vi "ROI and SWC editing tool.vi"() -> ()   [LabVIEW 2017]
panel:
  in  "Stop Button":bool
  in  "Open ROI data file":bool
  in  "Tab Control":T1(tab)
  in  "ROI":i32(listbox)
  in  "SWC":i32(listbox)
  out "ROI.dat file":path
  out "SWC File":path
  out "ROI":string[][](array[string])
  out "error out":errorcluster
  in  "error in":errorcluster
  in  "file path (use dialog)":path
  in  "Top rows to delete":i32=5
  out "number":dbl[][](array[numeric])
  out "x-y":dbl[](array[numeric])
  out "dmotorZ":dbl[](array[numeric])
  out "daolZ":dbl[](array[numeric])
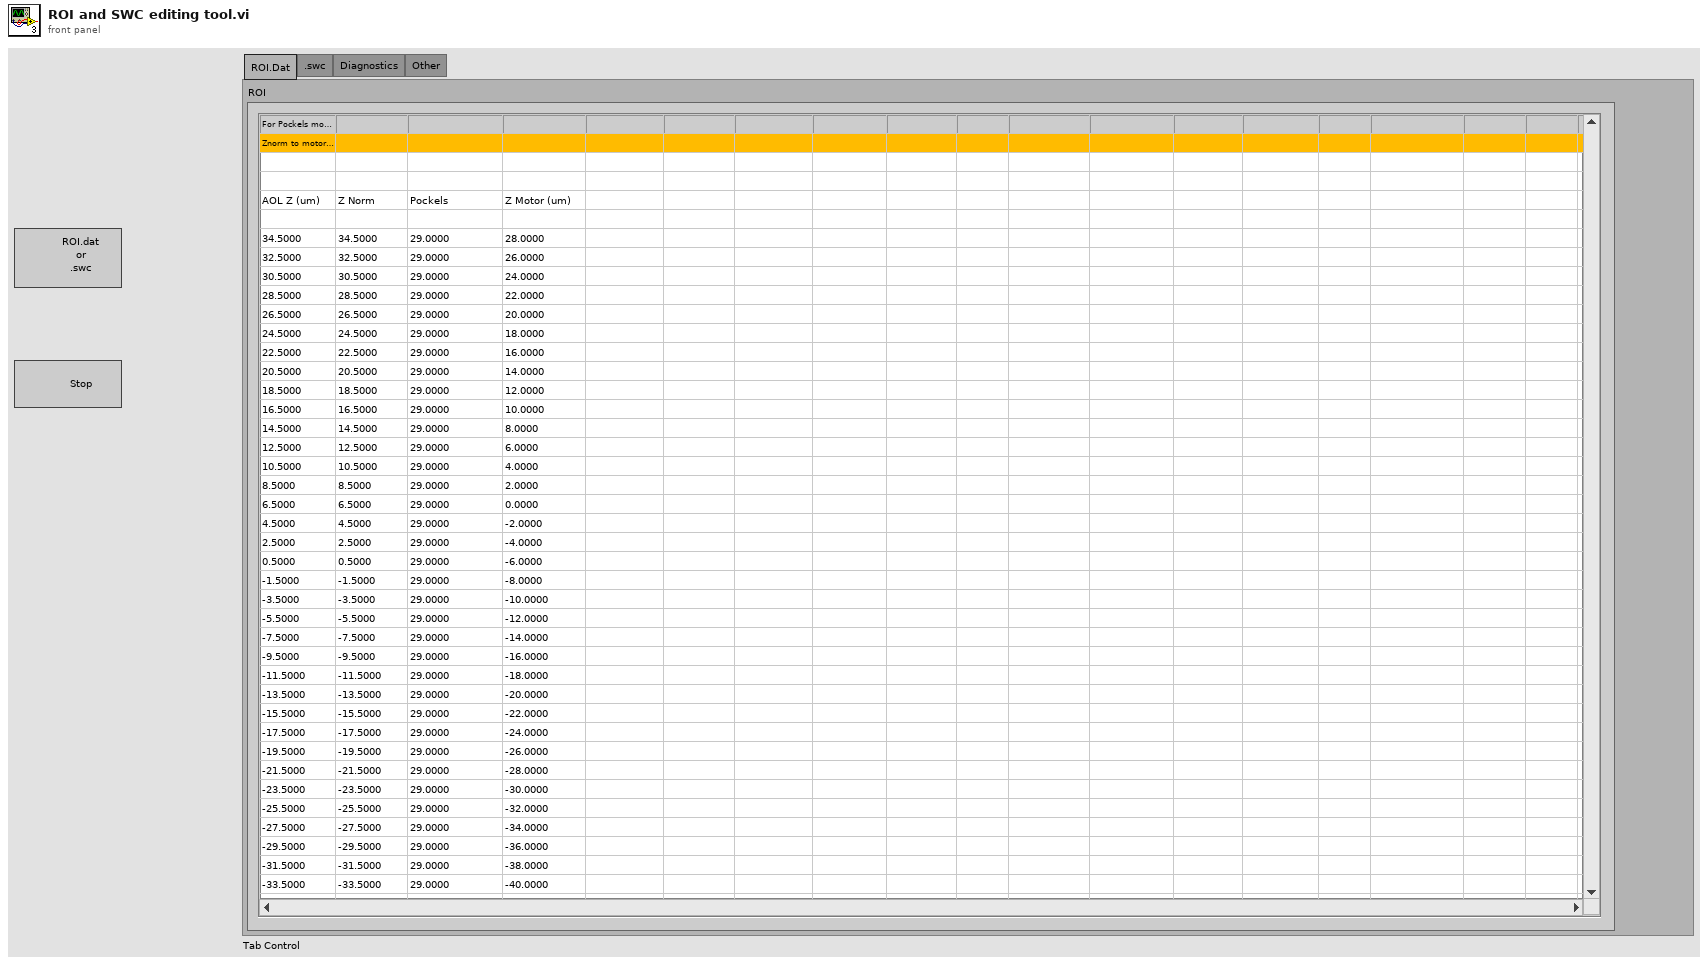
[diagram p1: front panel]
types:
  T1 = enum32{"ROI.Dat", ".swc", "Diagnostics", "Other"}
  T2 = enum16{"open", "replace", "create", "open or create", "replace or create", "replace or create with confirmation"}
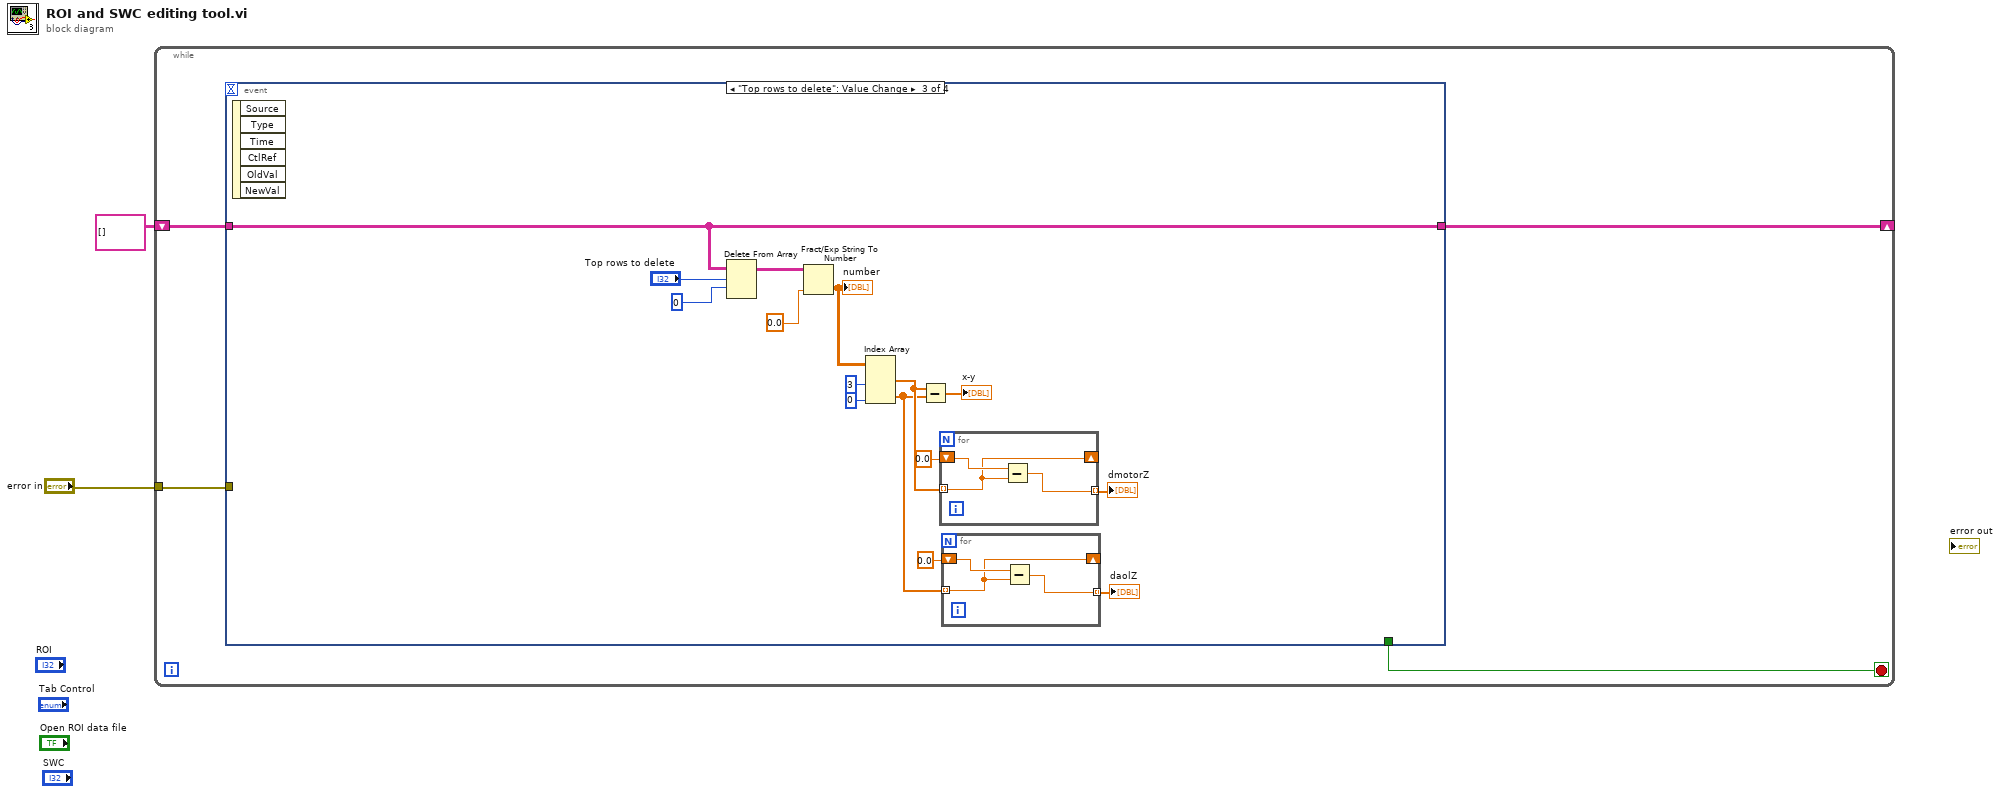
[diagram p0: block diagram]
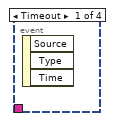
[diagram p2: hidden frame]
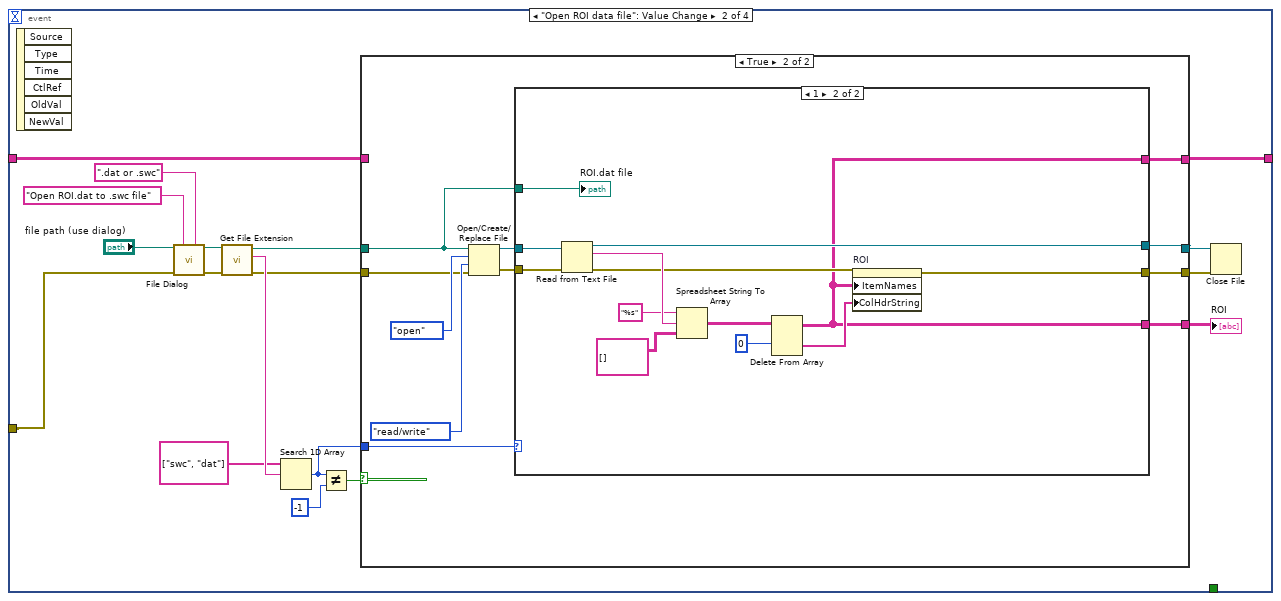
[diagram p3: hidden frame]
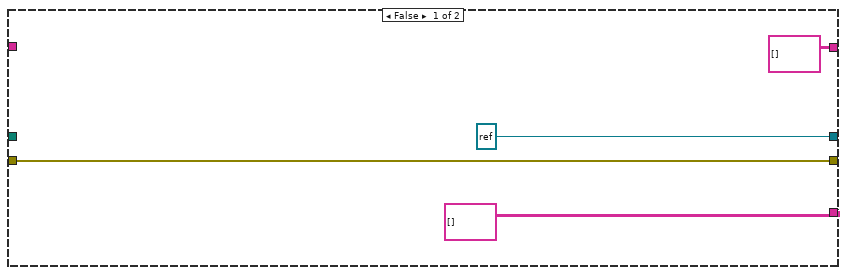
[diagram p4: hidden frame]
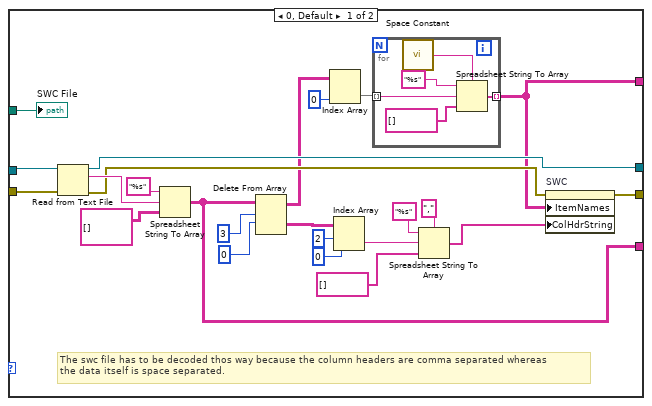
[diagram p5: hidden frame]
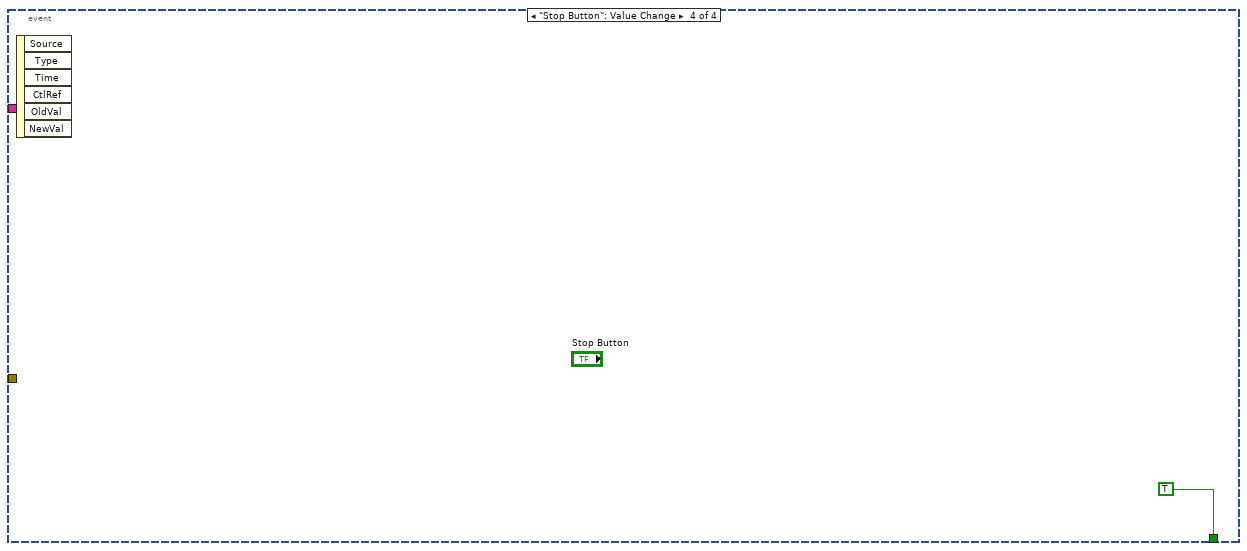
[diagram p6: hidden frame]
diagram:
  n1 = while {
    tunnel: "error in" -> [w6]
    shift-right: [w4] -> _
    shift-left: string[][] [] -> [w3]
    stop <- w5 stop-if-true
    n2 = event shown="[2] \"Top rows to delete\": Value Change" {
      selector: _ -> [_ _ _ _]
      dyn-events: _ -> [_ _ _ _]
      timeout: _ -> [_ _ _ _]
      tunnel: w6 -> [_ w9 _ _]
      tunnel: [_ _ _ TRUE] -> w5
      tunnel: [_ w8 w93 _] -> w4
      tunnel: w3 -> [_ w7 w93 _]
      event Timeout {
        n3 = event-data() -> ()  [unwired: 1 in, 3 out]
      }
      event "Open ROI data file": Value Change {
        n4 = event-data() -> ()  [unwired: 1 in, 6 out]
        n5 = call "File Dialog"("start path"="file path (use dialog)", "prompt"="Open ROI.dat to .swc file", "button label"=".dat or .swc" ("prompt"), "error in"=w9) -> ("selected path"=w16:path, "error out"=w15:errorcluster)  [unwired: 8 in, 2 out]
        n6 = call <vilib>:"Get File Extension.vi"("error in (no error)"=w15, "file"=w16) -> ("error out"=w17:errorcluster, "lowercase file extension"=w22:string, "dup file"=w18:path)  [unwired: 5 in, 2 out]
        n7 = Search 1D Array(1D array=string[] ["swc", "dat"], element=w22) -> (index of element=w24:i32)  [unwired: 1 in]
        n8 = Not Equal?(x=w24, y=-1) -> (x != y?=w23:bool)
        n9 = case shown="True" w23 {
          tunnel: w17 -> [w27 w37]
          tunnel: w18 -> [_ w30]
          tunnel: [string[][] [] w36] -> w19
          tunnel: [w27 w35] -> w20
          tunnel: [refnum<file> refnum ("refnum out") w31] -> w21
          tunnel: w24 -> [_ w34]
          tunnel: [string[][] [] w29] -> w8
          tunnel: w7 -> [_ _]
          frame False {
          }
          frame True {
            n10 = Open/Create/Replace File(file path (use dialog)=w30, error in=w37, operation (0:open)=T2."open", access (0:read/write)=enum16{"read/write", "read-only", "write-only"}."read/write") -> (refnum out=w32:refnum<file>, error out=w33:errorcluster)  [unwired: 2 in, 1 out]
            n11 = case shown="1" w34 {
              tunnel: [w48 w69] -> w36
              tunnel: [w63 w79] -> w35
              tunnel: w33 -> [w62 w75]
              tunnel: w32 -> [w61 w74]
              tunnel: [w49 w71] -> w31
              tunnel: w30 -> [w41 w70]
              tunnel: [w40 w69] -> w29
              frame 0, Default {
                # "The swc file has to be decoded thos way because the column headers are comma separated whereas\nthe data itself is space separated."
                n12 = Read from Text File(file (use dialog)=w61, error in=w62) -> (refnum out=w49:refnum<file>, text=w59:string, error out=w50:errorcluster)  [unwired: 2 in, 1 out]
                n13 = Spreadsheet String To Array(format string="%s", spreadsheet string=w59, array type (2D Dbl)=string[][] []) -> (array=w48:string[][])  [unwired: 1 in]
                n14 = Delete From Array(array=w48, length=3, index (row)=0 ("index")) -> (deleted portion=w55:string[][], array with subset deleted=w44:string[][])  [unwired: 1 in]
                n15 = Index Array(array=w44, index (col)=0 ("disabled index (col)")) -> (element=w42:string[])  [unwired: 1 in]
                n16 = Index Array(array=w55, index (row)=2, index (col)=0 ("disabled index (col)")) -> (element=w47:string)
                n17 = for {
                  tunnel: w42 -> [w68] mode=indexing
                  tunnel: [w65] -> w40 mode=indexing
                  n18 = call <vilib>:"Space Constant.vi"() -> ("String"=w64:string)
                  n19 = Spreadsheet String To Array(delimiter (Tab)=w64, format string="%s", spreadsheet string=w68, array type (2D Dbl)=string[] []) -> (array=w65:string[])
                }
                n20 = Spreadsheet String To Array(delimiter (Tab)=",", format string="%s", spreadsheet string=w47, array type (2D Dbl)=string[] []) -> (array=w51:string[])
                n21 = property on="SWC" class="MCListbox (strict)"(error in=w50, "ItemNames"=w40, "ColHdrString"=w51) -> (error out=w63:errorcluster)  [unwired: 1 in, 1 out]
                "SWC File" <- w41
              }
              frame 1 {
                n22 = Read from Text File(file (use dialog)=w74, error in=w75) -> (refnum out=w71:refnum<file>, text=w78:string, error out=w72:errorcluster)  [unwired: 2 in, 1 out]
                n23 = Spreadsheet String To Array(format string="%s", spreadsheet string=w78, array type (2D Dbl)=string[][] []) -> (array=w73:string[][])  [unwired: 1 in]
                n24 = Delete From Array(array=w73, index (row)=0) -> (deleted portion=w80:string[], array with subset deleted=w69:string[][])  [unwired: 2 in]
                n25 = property on="ROI" class="MCListbox (strict)"(error in=w72, "ItemNames"=w69, "ColHdrString"=w80) -> (error out=w79:errorcluster)  [unwired: 1 in, 1 out]
                "ROI.dat file" <- w70
              }
            }
          }
        }
        "ROI" <- w19
        n26 = Close File(refnum=w21, error in=w20) -> ()  [unwired: 2 out]
      }
      event "Top rows to delete": Value Change {
        n27 = event-data() -> ()  [unwired: 1 in, 6 out]
        n28 = Delete From Array(array=w93, length="Top rows to delete", index (row)=0) -> (array with subset deleted=w96:string[][])  [unwired: 1 in, 1 out]
        n29 = Fract/Exp String To Number(string=w96, default (0 dbl)=0.0) -> (number=w92:dbl[][])  [unwired: 2 in, 1 out]
        "number" <- w92
        n30 = Index Array(array=w92, index (col) #1=3 ("disabled index (col)"), index (col) #2=0 ("index (col)")) -> (element #1=w87:dbl[], element #2=w82:dbl[])  [unwired: 2 in]
        n31 = Subtract(x=w87, y=w82) -> (x-y=→"x-y":dbl[])
        n32 = for {
          tunnel: w87 -> [w100] mode=indexing
          shift-right: [w100] -> _
          shift-left: 0.0 -> [w102]
          tunnel: [w101] -> w85 mode=indexing
          n33 = Subtract(x=w102, y=w100) -> (x-y=w101:dbl)
        }
        "dmotorZ" <- w85
        n34 = for {
          tunnel: w82 -> [w97] mode=indexing
          shift-right: [w97] -> _
          shift-left: 0.0 -> [w99]
          tunnel: [w98] -> w84 mode=indexing
          n35 = Subtract(x=w99, y=w97) -> (x-y=w98:dbl)
        }
        "daolZ" <- w84
      }
      event "Stop Button": Value Change {
        n36 = event-data() -> ()  [unwired: 1 in, 6 out]
      }
    }
  }
